vi "AE Variables.vi"(0 "VariantIn":variant, 5 "error in (no error)":errorcluster, 8 "Action":T1=enum."Set Blue Pressure") -> (10 "Dbl Array":dbl[][](array[numeric]), 12 "Variant":variant, 14 "NumericOut":dbl, 15 "stringArray":string[](array[string]), 16 "BooleanOut":bool=TRUE, 17 "RingOut":u16(ring) items=["Hanning", "MA 5", "MA 8"], 18 "String":string, 19 "error out":errorcluster)   [LabVIEW 2013, in "main.lvlib"]
uses:
  main.lvlib
  Controls/Enum Variables.ctl
panel:
  in  "Excel._Application":refnum<k7>
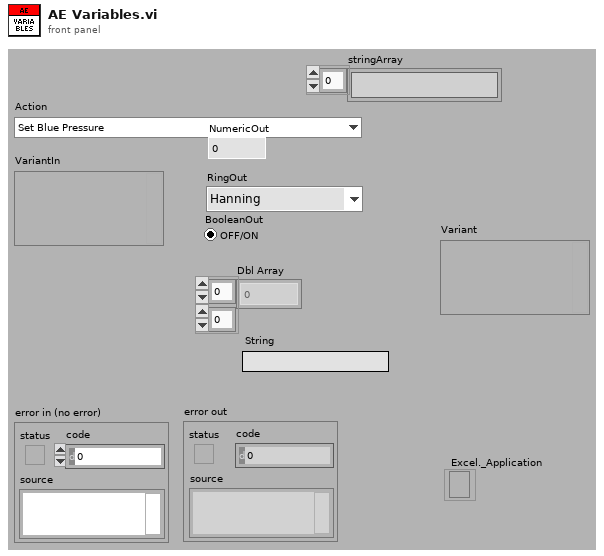
[diagram p1: front panel]
types:
  T1 = typedef "main.lvlib/Enum Variables.ctl" = enum16{"SetAcqFilter", "GetAcqFilter", "Set Filter", "Get Filter", "Set Height", "Get Height", "Set Recorded Height", "Get Recorded Height", "Set Blue Pressure", "Get Blue Pressure", "Set Red Pressure", "Get Red Pressure", "Init", "Reset Pressure", "Set Red Cursors", "Get Red Cursors", "Set Blue Cursors", "Get Blue Cursors", "Set Language", "Get Language", "Set Active Graphs", "Get ActiveGraphs", "Set Method", "Get Method", "Set Encryption", "Get Encryption", "Set ExcelVersion", "Get ExcelVersion", "Set DICOM Avail", "Get DICOM Avail", "Set DICOM Encode", "Get DICOM Encode", "Set JournalExport", "Get JournalExport", "Set Sequence", "Get Sequence", "Set DAQ Connected", "Get DAQ Connected", "Set Current Graph", "Get Current Graph", "Set General Settings", "Get Hyphenation", "Set Arm Calc Method", "Get Arm Calc Method", "Set Dicom Tags", "Get Dicom Tags", "Set BT Serial", "Get BT Serial", "Set BT Accepted Serials", "Get BT Accepted Serials", "Get BT License", "Set BT License"}
  T2 = cluster{"Red Pressure":dbl, "Blue Pressure":dbl, "Height":dbl, "AcqFilt":u16, "Filter":bool, "RedPositionArray":dbl[][], "BluePositionArray":dbl[][], "ActiveGraphs":u16, "Method":i32, "Encryption":bool, "ExcelVersion":i32, "DICOM Avail":bool, "DICOM Store Method":u16, "JournalType":u16, "Sequence":string, "DAQ Connected?":bool, "Current Graph":cluster{"Pressure":dbl[], "Graph":dbl[]}, "General Settings":cluster{"Hyphenation":bool, "Language":u16, "CellStr1":string, "CellStr2":string}, "ArmCalcMethod":dbl, "Dicom Tags":string[][], "BT Serial":cluster{"Serial Number":string, "Side":string, "Ignore?":bool}[], "BT Accepted Serials":string[], "BT License":string, "Recorded Height":i32}
  T3 = cluster{"Hyphenation":bool, "Language":u16, "CellStr1":string, "CellStr2":string}
  T4 = cluster{"Serial Number":string, "Side":string, "Ignore?":bool}[]
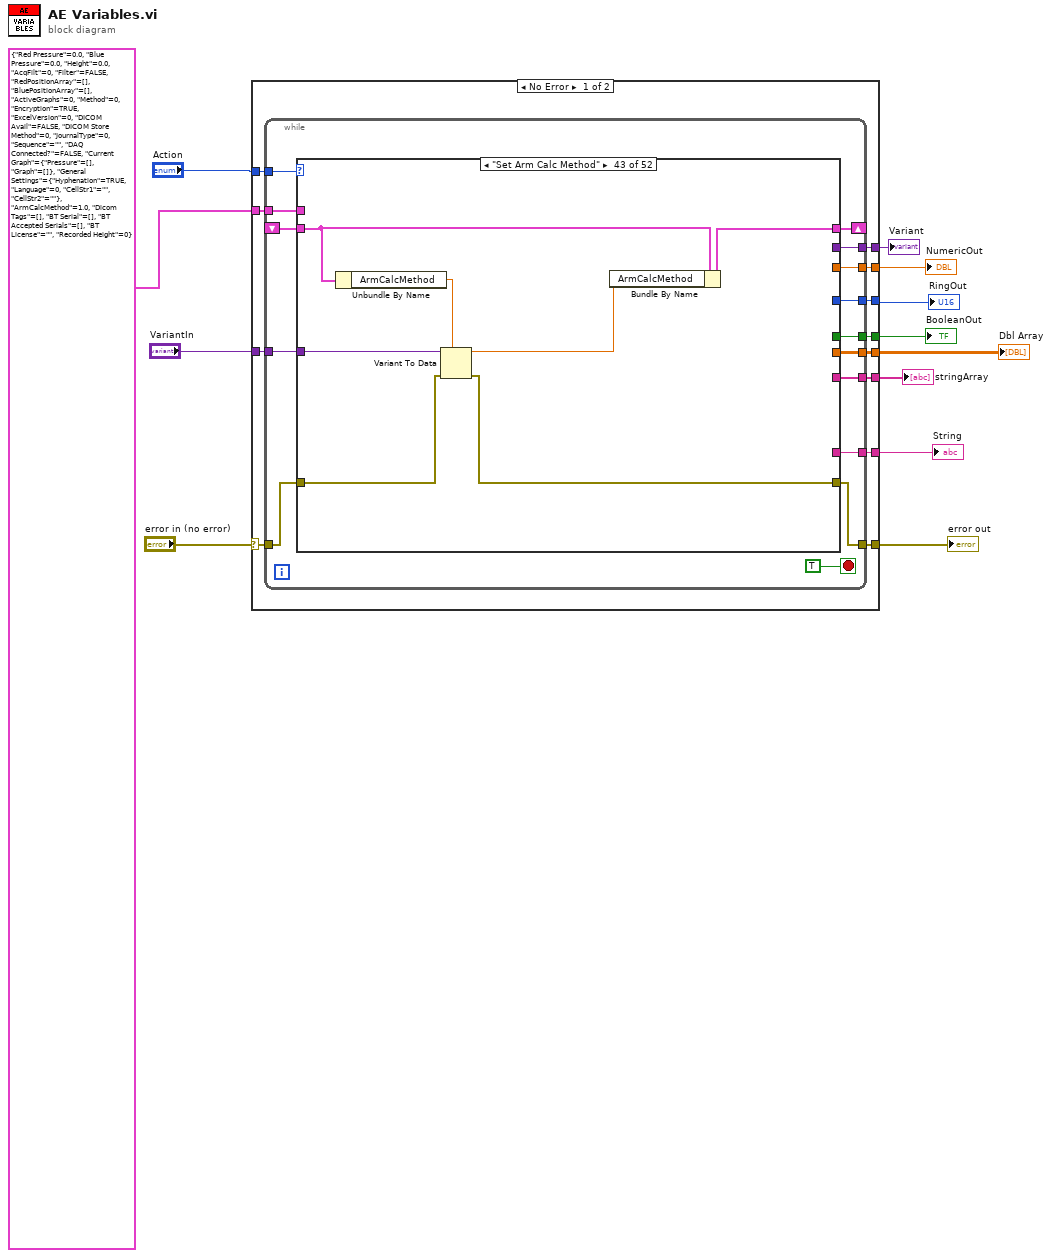
[diagram p0: block diagram]
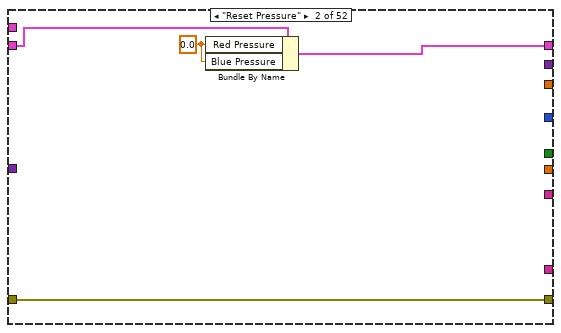
[diagram p3: hidden frame]
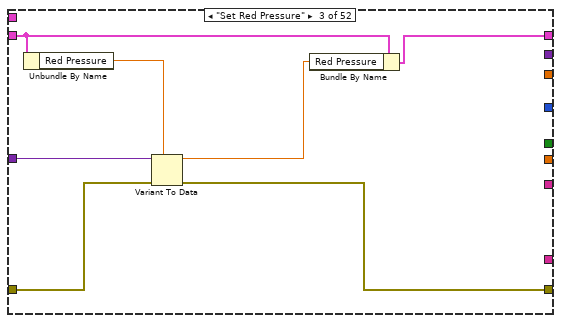
[diagram p4: hidden frame]
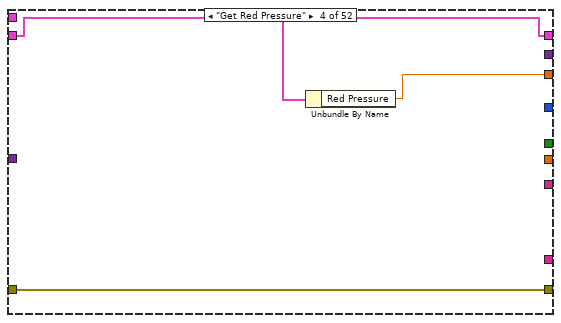
[diagram p5: hidden frame]
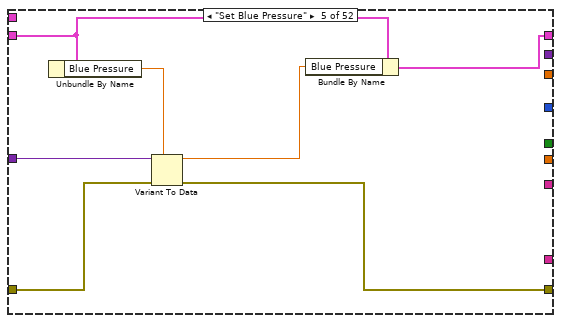
[diagram p6: hidden frame]
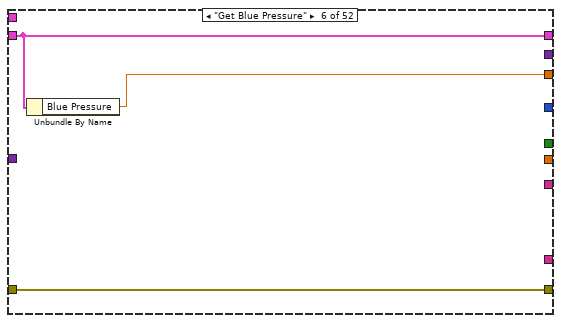
[diagram p7: hidden frame]
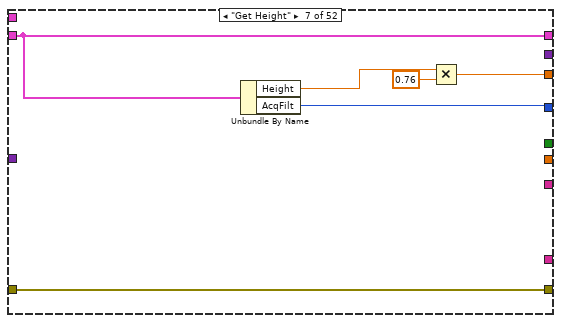
[diagram p8: hidden frame]
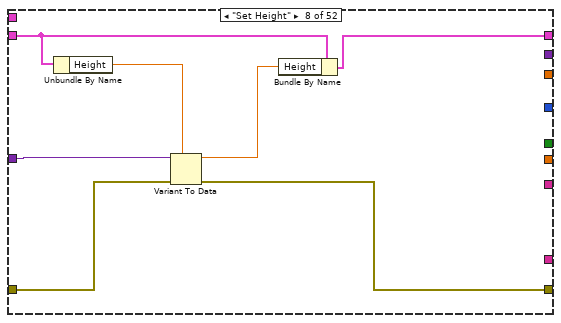
[diagram p9: hidden frame]
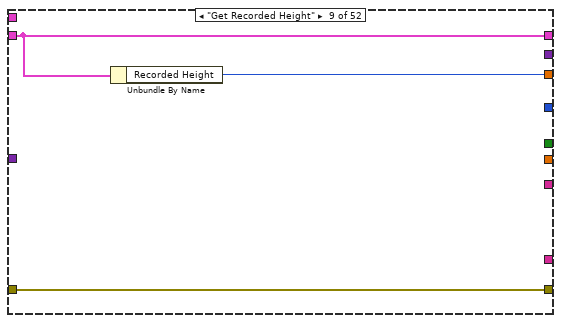
[diagram p10: hidden frame]
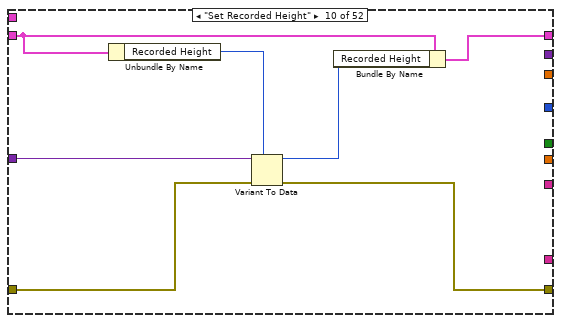
[diagram p11: hidden frame]
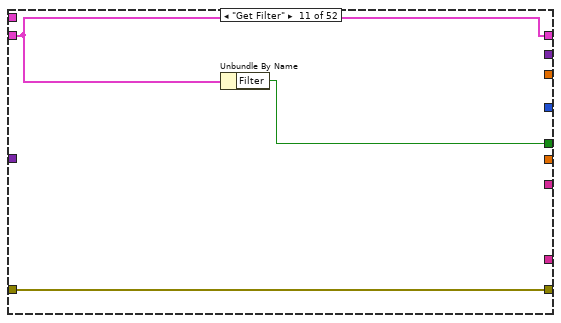
[diagram p12: hidden frame]
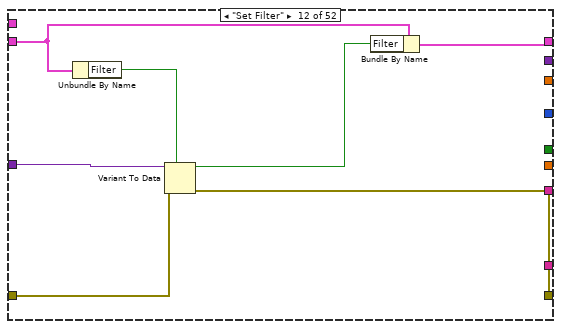
[diagram p13: hidden frame]
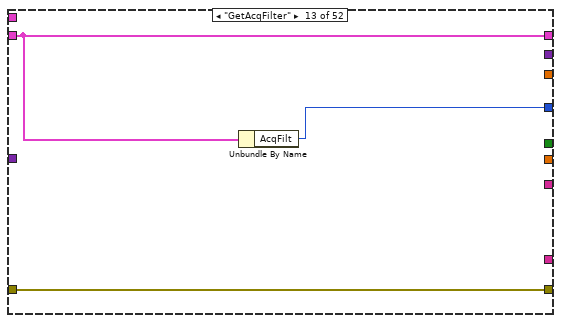
[diagram p14: hidden frame]
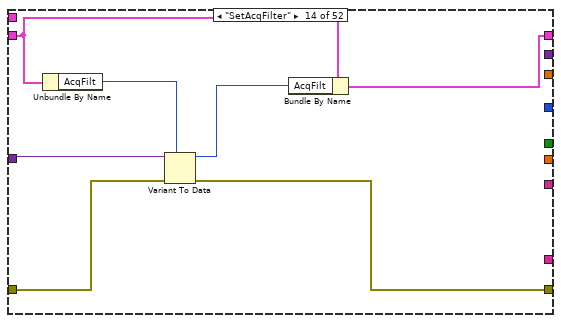
[diagram p15: hidden frame]
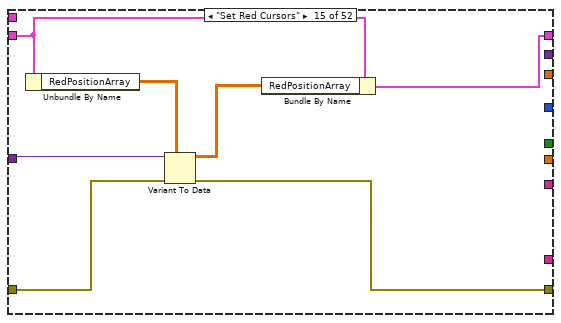
[diagram p16: hidden frame]
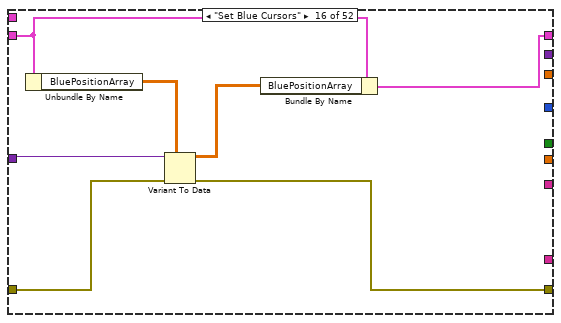
[diagram p17: hidden frame]
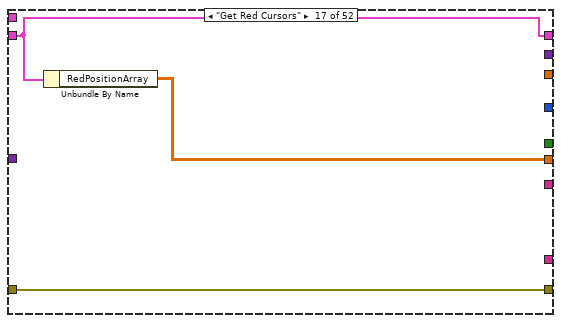
[diagram p18: hidden frame]
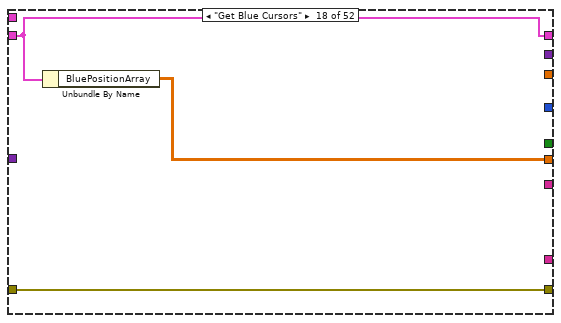
[diagram p19: hidden frame]
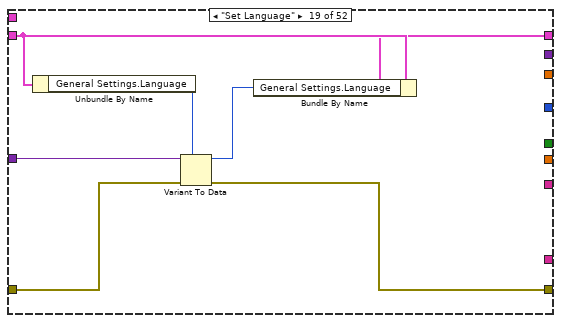
[diagram p20: hidden frame]
diagram:
  n1 = case shown="No Error" "error in (no error)" {
    selector: "error in (no error)" -> [w23 w316]
    tunnel: "Action" -> [w24 _]
    tunnel: [w22 w316] -> w11
    tunnel: "VariantIn" -> [w21 _]
    tunnel: T2 {"Red Pressure"=0.0, "Blue Pressure"=0.0, "Height"=0.0, "AcqFilt"=0, "Filter"=FALSE, "RedPositionArray"=[], "BluePositionArray"=[], "ActiveGraphs"=0, "Method"=0, "Encryption"=TRUE, "ExcelVersion"=0, "DICOM Avail"=FALSE, "DICOM Store Method"=0, "JournalType"=0, "Sequence"="", "DAQ Connected?"=FALSE, "Current Graph"={"Pressure"=[], "Graph"=[]}, "General Settings"={"Hyphenation"=TRUE, "Language"=0, "CellStr1"="", "CellStr2"=""}, "ArmCalcMethod"=1.0, "Dicom Tags"=[], "BT Serial"=[], "BT Accepted Serials"=[], "BT License"="", "Recorded Height"=0} -> [w20 _]
    tunnel: [w19 _] -> w7
    tunnel: [w18 _] -> w6
    tunnel: [w17 _] -> w5
    tunnel: [w16 _] -> w4
    tunnel: [w15 _] -> w3
    tunnel: [w14 _] -> w2
    tunnel: [w13 _] -> w1
    frame No Error {
      n2 = while {
        tunnel: w24 -> [w39]
        tunnel: w23 -> [w32]
        tunnel: [w31] -> w22
        tunnel: w21 -> [w37]
        shift-right: [w36] -> _
        shift-left: _ -> [w30]
        tunnel: w20 -> [w29]
        tunnel: [w35] -> w19
        tunnel: [w34] -> w18
        tunnel: [w33] -> w17
        tunnel: [w28] -> w16
        tunnel: [w27] -> w15
        tunnel: [w26] -> w14
        tunnel: [w25] -> w13
        stop <- TRUE stop-if-true
        n3 = case shown="\"Set Arm Calc Method\"" w39 {
          tunnel: w37 -> [_ _ w51 _ w60 _ _ w77 _ w83 _ w97 _ w107 w114 w121 _ _ w133 _ w143 _ w155 _ w165 _ _ _ w195 _ w205 _ w215 _ w226 _ w236 _ w244 _ w255 _ w270 _ w280 _ w288 _ w298 _ w310 _]
          tunnel: [w40 w45 w52 w53 w62 w63 w66 w78 w79 w86 w89 w98 w99 w108 w115 w122 w125 w128 w130 w136 w140 w148 w152 w158 w161 w167 w174 w187 w191 w198 w202 w206 w212 w219 w222 w232 w233 w242 w245 w253 w256 w263 w266 w273 w274 w284 w285 w295 w299 w305 w307 w315] -> w36
          tunnel: [_ _ _ w55 _ w64 w69 _ w81 _ _ _ _ _ _ _ _ _ _ _ _ _ _ w157 _ _ _ w188 _ _ _ _ _ _ _ _ _ _ _ _ _ _ _ w272 _ _ _ _ _ _ _ _] -> w35
          tunnel: [_ _ _ _ _ _ _ _ _ _ w91 _ _ _ _ _ _ _ _ _ _ _ _ _ _ w168 _ _ _ w197 _ _ _ _ _ _ _ w241 _ _ _ w262 _ _ _ _ _ _ _ _ _ _] -> w34
          tunnel: [_ _ _ _ _ _ w68 _ _ _ _ _ w101 _ _ _ _ _ _ w137 _ w147 _ _ _ _ _ _ _ _ _ w208 _ w221 _ _ _ _ _ _ _ _ _ _ _ _ _ _ _ _ _ _] -> w33
          tunnel: w32 -> [w41 w43 w49 w54 w58 w65 w67 w74 w80 w84 w90 w94 w100 w104 w111 w118 w124 w127 w132 w138 w142 w146 w149 w156 w164 w166 w176 w186 w194 w196 w204 w207 w214 w220 w225 w229 w235 w240 w247 w252 w258 w261 w269 w271 w279 w283 w287 w292 w297 w303 w309 w314]
          tunnel: [w41 w43 w48 w54 w57 w65 w67 w73 w80 w82 w90 w93 w100 w103 w110 w117 w124 w127 w129 w138 w139 w146 w150 w156 w163 w166 w171 w186 w189 w196 w200 w207 w210 w220 w224 w229 w234 w240 w243 w252 w254 w261 w264 w271 w277 w283 w286 w292 w296 w303 w306 w314] -> w31
          tunnel: w30 -> [_ w42 w46 w53 w56 w63 w66 w72 w79 w85 w89 w92 w99 w102 w109 w116 w125 w128 w131 w136 w141 w148 w153 w158 w160 w167 w175 w187 w192 w198 w199 w206 w209 w219 w223 w232 w237 w242 w246 w253 w257 w263 w267 w273 w276 w284 w289 w295 w300 w305 w308 w315]
          tunnel: w29 -> [w40 _ _ _ _ _ _ _ _ _ _ _ _ _ _ _ _ _ _ _ _ _ _ _ _ _ _ _ _ _ _ _ _ _ _ _ _ _ _ _ _ _ _ _ _ _ _ _ _ _ _ _]
          tunnel: [_ _ _ _ _ _ _ _ _ _ _ _ _ _ _ _ w123 w126 _ _ _ _ _ _ _ _ _ _ _ _ _ _ _ _ _ _ _ _ _ _ _ _ _ _ _ _ _ _ _ _ _ _] -> w28
          tunnel: [_ _ _ _ _ _ _ _ _ _ _ _ _ _ _ _ _ _ _ _ _ _ _ _ _ _ _ _ _ _ _ _ _ w216 _ w230 _ _ _ _ _ _ _ _ _ _ _ _ _ w304 _ _] -> w27
          tunnel: [_ _ _ _ _ _ _ _ _ _ _ _ _ _ _ _ _ _ _ _ _ _ _ _ _ _ _ _ _ _ _ _ _ _ _ _ _ _ _ w251 _ _ _ _ _ w281 _ w294 _ _ _ _] -> w26
          tunnel: [_ _ _ _ _ _ _ _ _ _ _ _ _ _ _ _ _ _ _ _ _ _ _ _ _ _ _ _ _ _ _ _ _ _ _ _ _ _ _ _ _ _ _ _ _ _ _ _ _ _ _ w313] -> w25
          frame "Init", Default {
          }
          frame "Reset Pressure" {
            w44 = 0.0 ("Red Pressure")
            n4 = Bundle By Name(cluster=w42, "Red Pressure"=w44, "Blue Pressure"=w44) -> (w45:T2)
          }
          frame "Set Red Pressure" {
            n5 = Unbundle By Name(w46) -> ("Red Pressure"=w47:dbl)
            n6 = Variant To Data(error in=w49, type=w47, Variant=w51) -> (data=w50:dbl, error out=w48:errorcluster)
            n7 = Bundle By Name(cluster=w46, "Red Pressure"=w50) -> (w52:T2)
          }
          frame "Get Red Pressure" {
            n8 = Unbundle By Name(w53) -> ("Red Pressure"=w55:dbl)
          }
          frame "Set Blue Pressure" {
            n9 = Unbundle By Name(w56) -> ("Blue Pressure"=w61:dbl)
            n10 = Variant To Data(error in=w58, type=w61, Variant=w60) -> (data=w59:dbl, error out=w57:errorcluster)
            n11 = Bundle By Name(cluster=w56, "Blue Pressure"=w59) -> (w62:T2)
          }
          frame "Get Blue Pressure" {
            n12 = Unbundle By Name(w63) -> ("Blue Pressure"=w64:dbl)
          }
          frame "Get Height" {
            n13 = Unbundle By Name(w66) -> ("Height"=w70:dbl, "AcqFilt"=w68:u16)
            n14 = Multiply(x=w70, y=0.76) -> (x*y=w69:dbl)
          }
          frame "Set Height" {
            n15 = Unbundle By Name(w72) -> ("Height"=w76:dbl)
            n16 = Variant To Data(error in=w74, type=w76, Variant=w77) -> (data=w75:dbl, error out=w73:errorcluster)
            n17 = Bundle By Name(cluster=w72, "Height"=w75) -> (w78:T2)
          }
          frame "Get Recorded Height" {
            n18 = Unbundle By Name(w79) -> ("Recorded Height"=w81:i32)
          }
          frame "Set Recorded Height" {
            n19 = Unbundle By Name(w85) -> ("Recorded Height"=w88:i32)
            n20 = Variant To Data(error in=w84, type=w88, Variant=w83) -> (data=w87:i32, error out=w82:errorcluster)
            n21 = Bundle By Name(cluster=w85, "Recorded Height"=w87) -> (w86:T2)
          }
          frame "Get Filter" {
            n22 = Unbundle By Name(w89) -> ("Filter"=w91:bool)
          }
          frame "Set Filter" {
            n23 = Unbundle By Name(w92) -> ("Filter"=w96:bool)
            n24 = Variant To Data(error in=w94, type=w96, Variant=w97) -> (data=w95:bool, error out=w93:errorcluster)
            n25 = Bundle By Name(cluster=w92, "Filter"=w95) -> (w98:T2)
          }
          frame "GetAcqFilter" {
            n26 = Unbundle By Name(w99) -> ("AcqFilt"=w101:u16)
          }
          frame "SetAcqFilter" {
            n27 = Unbundle By Name(w102) -> ("AcqFilt"=w105:u16)
            n28 = Variant To Data(error in=w104, type=w105, Variant=w107) -> (data=w106:u16, error out=w103:errorcluster)
            n29 = Bundle By Name(cluster=w102, "AcqFilt"=w106) -> (w108:T2)
          }
          frame "Set Red Cursors" {
            n30 = Unbundle By Name(w109) -> ("RedPositionArray"=w112:dbl[][])
            n31 = Variant To Data(error in=w111, type=w112, Variant=w114) -> (data=w113:dbl[][], error out=w110:errorcluster)
            n32 = Bundle By Name(cluster=w109, "RedPositionArray"=w113) -> (w115:T2)
          }
          frame "Set Blue Cursors" {
            n33 = Unbundle By Name(w116) -> ("BluePositionArray"=w119:dbl[][])
            n34 = Variant To Data(error in=w118, type=w119, Variant=w121) -> (data=w120:dbl[][], error out=w117:errorcluster)
            n35 = Bundle By Name(cluster=w116, "BluePositionArray"=w120) -> (w122:T2)
          }
          frame "Get Red Cursors" {
            n36 = Unbundle By Name(w125) -> ("RedPositionArray"=w123:dbl[][])
          }
          frame "Get Blue Cursors" {
            n37 = Unbundle By Name(w128) -> ("BluePositionArray"=w126:dbl[][])
          }
          frame "Set Language" {
            n38 = Unbundle By Name(w131) -> ("General Settings.Language"=w134:u16)
            n39 = Variant To Data(error in=w132, type=w134, Variant=w133) -> (data=w135:u16, error out=w129:errorcluster)
            n40 = Bundle By Name(cluster=w131, "General Settings.Language"=w135) -> (w130:T2)
          }
          frame "Get Language" {
            n41 = Unbundle By Name(w136) -> ("General Settings.Language"=w137:u16)
          }
          frame "Set Active Graphs" {
            n42 = Unbundle By Name(w141) -> ("ActiveGraphs"=w144:u16)
            n43 = Variant To Data(error in=w142, type=w144, Variant=w143) -> (data=w145:u16, error out=w139:errorcluster)
            n44 = Bundle By Name(cluster=w141, "ActiveGraphs"=w145) -> (w140:T2)
          }
          frame "Get ActiveGraphs" {
            n45 = Unbundle By Name(w148) -> ("ActiveGraphs"=w147:u16)
          }
          frame "Set Method" {
            n46 = Unbundle By Name(w153) -> ("Method"=w154:i32)
            n47 = Variant To Data(error in=w149, type=w154, Variant=w155) -> (data=w151:i32, error out=w150:errorcluster)
            n48 = Bundle By Name(cluster=w153, "Method"=w151) -> (w152:T2)
          }
          frame "Get Method" {
            n49 = Unbundle By Name(w158) -> ("Method"=w157:i32)
          }
          frame "Set Encryption" {
            n50 = Unbundle By Name(w160) -> ("Encryption"=w159:bool)
            n51 = Variant To Data(error in=w164, type=w159, Variant=w165) -> (data=w162:bool, error out=w163:errorcluster)
            n52 = Bundle By Name(cluster=w160, "Encryption"=w162) -> (w161:T2)
          }
          frame "Get Encryption" {
            n53 = Unbundle By Name(w167) -> ("Encryption"=w168:bool)
          }
          frame "Set ExcelVersion" {
            n54 = Automation Open(error in (no error)=w176, Automation Refnum="Excel._Application") -> (Automation Refnum=w173:refnum<k7>, error out=w178:errorcluster)  [unwired: 2 in]
            n55 = property class="_Application"(reference=w173, error in=w178) -> (reference out=w179:refnum<k7>, error out=w177:errorcluster, "Version"=w170:string)
            n56 = Close Reference(reference=w179, error in (no error)=w177) -> (error out=w172:errorcluster)
            n57 = case shown="No Error" w172 {
              selector: w172 -> [w183 _]
              tunnel: [w183 errorcluster {"status"=FALSE, "code"=0, "source"=""} ("error IO")] -> w171
              tunnel: w170 -> [w182 _]
              tunnel: [w181 11] -> w169
              frame No Error {
                n58 = Decimal String To Number(string=w182) -> (number=w181:i32)  [unwired: 2 in, 1 out]
              }
              frame Error {
              }
            }
            n59 = Bundle By Name(cluster=w175, "ExcelVersion"=w169) -> (w174:T2)
          }
          frame "Get ExcelVersion" {
            n60 = Unbundle By Name(w187) -> ("ExcelVersion"=w188:i32)
          }
          frame "Set DICOM Avail" {
            n61 = Unbundle By Name(w192) -> ("DICOM Avail"=w193:bool)
            n62 = Variant To Data(error in=w194, type=w193, Variant=w195) -> (data=w190:bool, error out=w189:errorcluster)
            n63 = Bundle By Name(cluster=w192, "DICOM Avail"=w190) -> (w191:T2)
          }
          frame "Get DICOM Avail" {
            n64 = Unbundle By Name(w198) -> ("DICOM Avail"=w197:bool)
          }
          frame "Set DICOM Encode" {
            n65 = Unbundle By Name(w199) -> ("DICOM Store Method"=w203:u16)
            n66 = Variant To Data(error in=w204, type=w203, Variant=w205) -> (data=w201:u16, error out=w200:errorcluster)
            n67 = Bundle By Name(cluster=w199, "DICOM Store Method"=w201) -> (w202:T2)
          }
          frame "Get DICOM Encode" {
            n68 = Unbundle By Name(w206) -> ("DICOM Store Method"=w208:u16)
          }
          frame "Set JournalExport" {
            n69 = Unbundle By Name(w209) -> ("JournalType"=w213:u16)
            n70 = Variant To Data(error in=w214, type=w213, Variant=w215) -> (data=w211:u16, error out=w210:errorcluster)
            n71 = Bundle By Name(cluster=w209, "JournalType"=w211) -> (w212:T2)
          }
          frame "Get JournalExport" {
            n72 = Unbundle By Name(w219) -> ("JournalType"=w221:u16, "General Settings.CellStr1"=w218:string, "General Settings.CellStr2"=w217:string)
            n73 = Build Array(w218, w217) -> (w216:string[])
          }
          frame "Set Sequence" {
            n74 = Unbundle By Name(w223) -> ("Sequence"=w227:string)
            n75 = Variant To Data(error in=w225, type=w227, Variant=w226) -> (data=w228:string, error out=w224:errorcluster)
            n76 = Bundle By Name(cluster=w223, "Sequence"=w228) -> (w222:T2)
          }
          frame "Get Sequence" {
            n77 = Unbundle By Name(w232) -> ("Sequence"=w231:string)
            n78 = Build Array(w231) -> (w230:string[])
          }
          frame "Set DAQ Connected" {
            n79 = Unbundle By Name(w237) -> ("DAQ Connected?"=w238:bool)
            n80 = Variant To Data(error in=w235, type=w238, Variant=w236) -> (data=w239:bool, error out=w234:errorcluster)
            n81 = Bundle By Name(cluster=w237, "DAQ Connected?"=w239) -> (w233:T2)
          }
          frame "Get DAQ Connected" {
            n82 = Unbundle By Name(w242) -> ("DAQ Connected?"=w241:bool)
          }
          frame "Set Current Graph" {
            n83 = Unbundle By Name(w246) -> ("Current Graph"=w248:cluster{"Pressure":dbl[], "Graph":dbl[]})
            n84 = Variant To Data(error in=w247, type=w248, Variant=w244) -> (data=w249:cluster{"Pressure":dbl[], "Graph":dbl[]}, error out=w243:errorcluster)
            n85 = Bundle By Name(cluster=w246, "Current Graph"=w249) -> (w245:T2)
          }
          frame "Get Current Graph" {
            n86 = Unbundle By Name(w253) -> ("Current Graph"=w250:cluster{"Pressure":dbl[], "Graph":dbl[]})
            n87 = To Variant(anything=w250) -> (Variant=w251:variant)
          }
          frame "Set General Settings" {
            n88 = Unbundle By Name(w257) -> ("General Settings"=w259:T3)
            n89 = Variant To Data(error in=w258, type=w259, Variant=w255) -> (data=w260:T3, error out=w254:errorcluster)
            n90 = Bundle By Name(cluster=w257, "General Settings"=w260) -> (w256:T2)
          }
          frame "Get Hyphenation" {
            n91 = Unbundle By Name(w263) -> ("General Settings.Hyphenation"=w262:bool)
          }
          frame "Set Arm Calc Method" {
            n92 = Unbundle By Name(w267) -> ("ArmCalcMethod"=w268:dbl)
            n93 = Variant To Data(error in=w269, type=w268, Variant=w270) -> (data=w265:dbl, error out=w264:errorcluster)
            n94 = Bundle By Name(cluster=w267, "ArmCalcMethod"=w265) -> (w266:T2)
          }
          frame "Get Arm Calc Method" {
            n95 = Unbundle By Name(w273) -> ("ArmCalcMethod"=w272:dbl)
          }
          frame "Set Dicom Tags" {
            n96 = Unbundle By Name(w276) -> ("Dicom Tags"=w278:string[][])
            n97 = Variant To Data(error in=w279, type=w278, Variant=w280) -> (data=w275:string[][], error out=w277:errorcluster)
            n98 = Bundle By Name(cluster=w276, "Dicom Tags"=w275) -> (w274:T2)
          }
          frame "Get Dicom Tags" {
            n99 = Unbundle By Name(w284) -> ("Dicom Tags"=w282:string[][])
            n100 = To Variant(anything=w282) -> (Variant=w281:variant)
          }
          frame "Set BT Serial" {
            n101 = Unbundle By Name(w289) -> ("BT Serial"=w291:T4)
            n102 = Variant To Data(error in=w287, type=w291, Variant=w288) -> (data=w290:T4, error out=w286:errorcluster)
            n103 = Bundle By Name(cluster=w289, "BT Serial"=w290) -> (w285:T2)
          }
          frame "Get BT Serial" {
            n104 = Unbundle By Name(w295) -> ("BT Serial"=w293:T4)
            n105 = To Variant(anything=w293) -> (Variant=w294:variant)
          }
          frame "Set BT Accepted Serials" {
            n106 = Unbundle By Name(w300) -> ("BT Accepted Serials"=w302:string[])
            n107 = Variant To Data(error in=w297, type=w302, Variant=w298) -> (data=w301:string[], error out=w296:errorcluster)
            n108 = Bundle By Name(cluster=w300, "BT Accepted Serials"=w301) -> (w299:T2)
          }
          frame "Get BT Accepted Serials" {
            n109 = Unbundle By Name(w305) -> ("BT Accepted Serials"=w304:string[])
          }
          frame "Set BT License" {
            n110 = Unbundle By Name(w308) -> ("BT License"=w312:string)
            n111 = Variant To Data(error in=w309, type=w312, Variant=w310) -> (data=w311:string, error out=w306:errorcluster)
            n112 = Bundle By Name(cluster=w308, "BT License"=w311) -> (w307:T2)
          }
          frame "Get BT License" {
            n113 = Unbundle By Name(w315) -> ("BT License"=w313:string)
          }
        }
      }
    }
    frame Error {
    }
  }
  "error out" <- w11
  "NumericOut" <- w7
  "BooleanOut" <- w6
  "RingOut" <- w5
  "Dbl Array" <- w4
  "stringArray" <- w3
  "Variant" <- w2
  "String" <- w1
